vi "Measure Image.vi"(0 "ROI Descriptors (Measure 1)":T1(array[cluster])=[{"Global Rectangle"=[1660, 520, 2246, 531], "Contours"=[{"ID"=enum."External", "Type"=2, "Coordinates"=[1660, 520, 2245, 530]}]}] {"Contours"."Type" items=["No Selection", "Point", "Line", "Rectangle", "Oval", "Polygon", "Freehand Region", "Annulus", "Unused2", "Unused3", "Broken Line", "Freehand Line", "Rotated Rectangle"]}, 1 "Measurements (Measure 1)":i32[](array[numeric])=[1], 7 "error in":errorcluster) -> (20 "Results (Measure 1)":string[][](array[string]), 27 "error out":errorcluster)   [LabVIEW 2016]
panel:
  out "Image Out":T2(plugin-control)
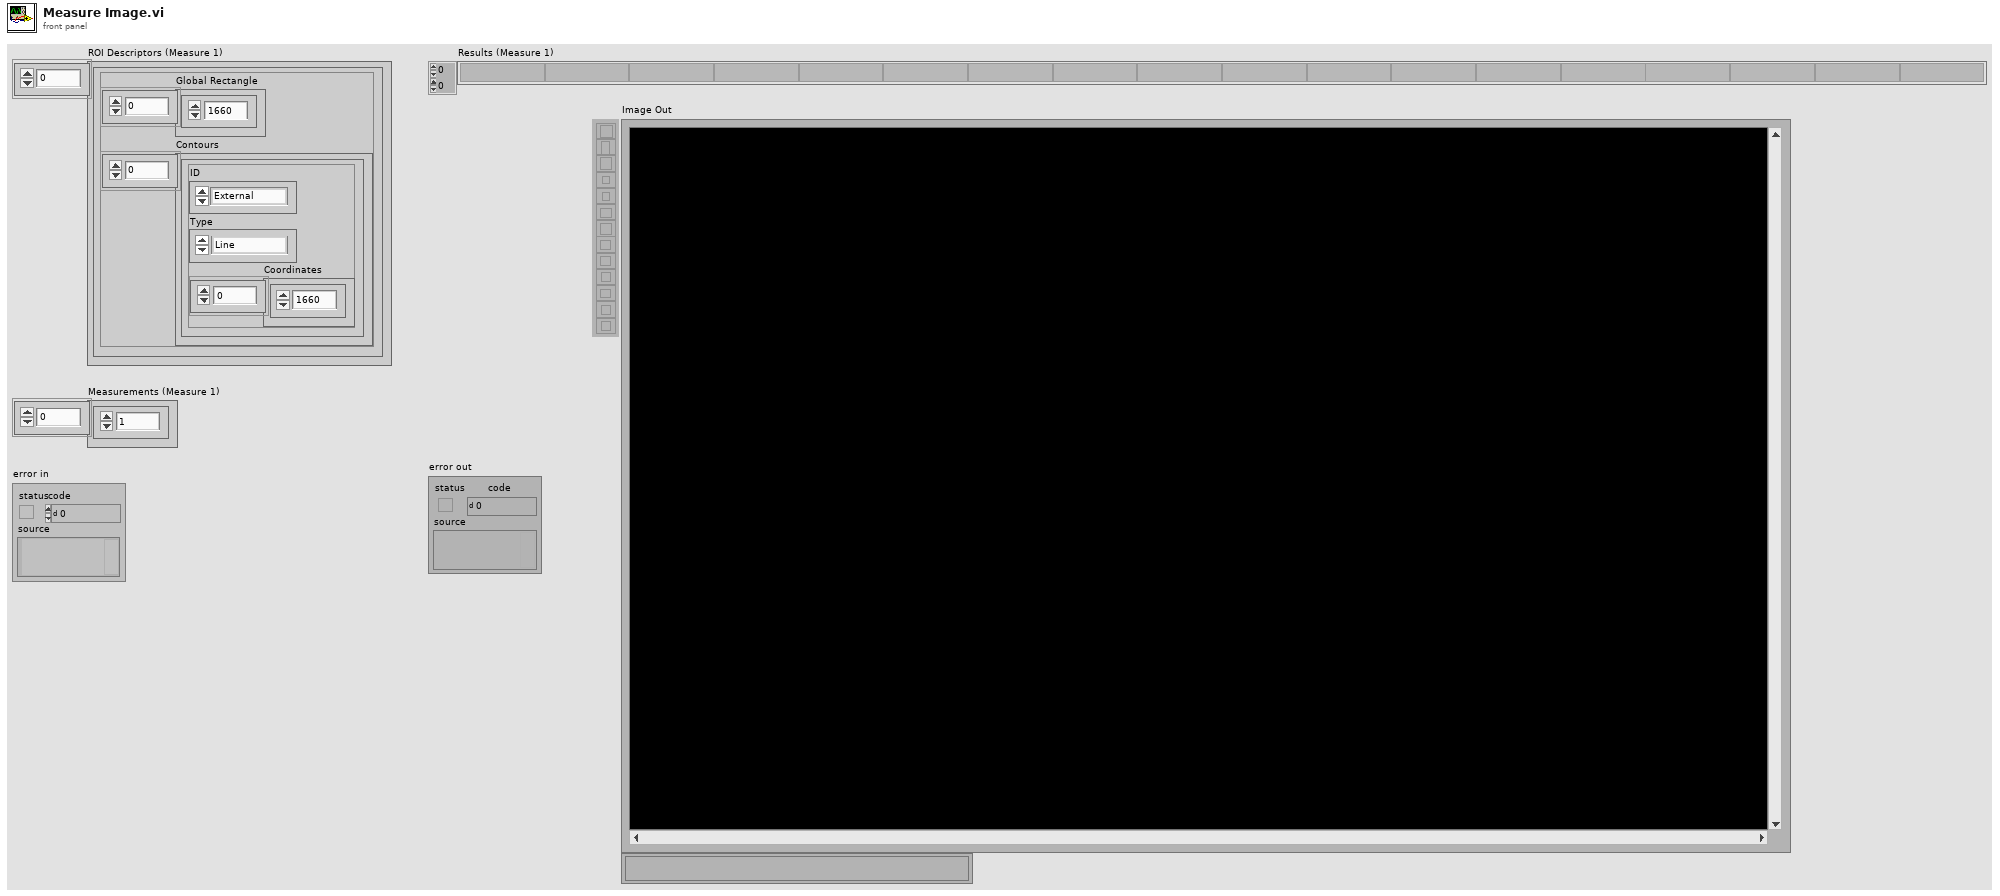
[diagram p1: front panel]
types:
  T1 = cluster{"Global Rectangle":i32[], "Contours":cluster{"ID":enum32{"External", "Internal"}, "Type":u32, "Coordinates":i32[]}[]}[]
  T2 = typedef "IMAQ Image.ctl" = refnum<image>
  T3 = typedef "Image Type" = u32
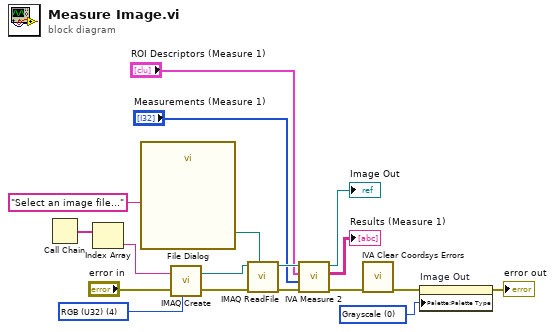
[diagram p0: block diagram]
diagram:
  w1 = u32 0 items=["Grayscale", "Binary", "Gradient", "Rainbow", "Temperature", "User Defined", "Binary 16 Bit", "Gradient 16 Bit", "Rainbow 16 Bit", "Temperature 16 Bit", "User Defined 16 Bit"] ("Palette Type")
  w10 = T3 4 items=["Grayscale (U8)", "Grayscale (I16)", "Grayscale (SGL)", "Complex (CSG)", "RGB (U32)", "HSL (U32)", "RGB (U64)", "Grayscale (U16)"] ("Image Type")
  n1 = Call Chain() -> (call chain=w14:string[])
  n2 = Index Array(array=w14) -> (element=w13:string)  [unwired: 1 in]
  n3 = call "File Dialog"("prompt"="Select an image file...") -> ("selected path"=w11:path)  [unwired: 6 in, 8 out]
  n4 = call "IMAQ Create"("Image Name"=w13, "Image Type"=w10, "error in (no error)"="error in") -> ("New Image"=w17:T2, "error out"=w16:errorcluster)  [unwired: 1 in, 1 out]
  n5 = call "IMAQ ReadFile"("File Path"=w11, "error in (no error)"=w16, "Image"=w17) -> ("error out"=w18:errorcluster, "Image Out"=w9:T2)  [unwired: 2 in, 5 out]
  n6 = call <vilib>:"IVA Measure 2.vi"("error in (no error)"=w18, "Measurements"="Measurements (Measure 1)", "ROI Descriptors"="ROI Descriptors (Measure 1)", "Image In"=w9) -> ("error out"=w5:errorcluster, "Results"=→"Results (Measure 1)":string[][], "Image Out"=→"Image Out":T2)  [unwired: 1 in, 4 out]
  n7 = call <vilib>:"IVA Clear Coordsys Errors.vi"("error in (no error)"=w5) -> ("error out"=w4:errorcluster)  [unwired: 10 in]
  n8 = property on="Image Out" class="ImageControl"(error in=w4, "Palette:Palette Type"=w1) -> (error out=→"error out":errorcluster)  [unwired: 1 in, 1 out]
